vi "Generate File Name.vi"() -> (3 "file name":string)   [LabVIEW 2017, in "Logger.lvclass"]
uses:
  logger/Logger.lvclass
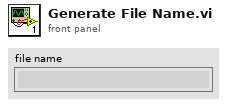
[diagram p1: front panel]
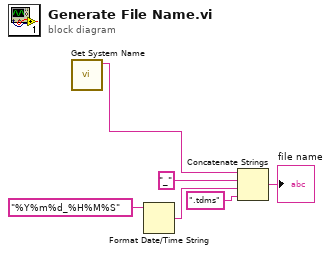
[diagram p0: block diagram]
diagram:
  n1 = call "Get System Name.vi"() -> ("name"=w2:string)  [unwired: 11 in]
  n2 = Format Date/Time String(time format string (%c)="%Y%m%d_%H%M%S") -> (date/time string=w3:string)  [unwired: 2 in]
  n3 = Concatenate Strings(w2, "_" ("string"), w3, ".tdms" ("string")) -> (→"file name":string)
